vi "GT Pvt Continuous Calculate.vi"(0 "cardNum":i16, 1 "n":i32, 2 "pPos":dbl, 3 "pVel":dbl, 4 "pPercent":dbl, 5 "pVelMax":dbl, 6 "pAcc":dbl, 7 "error in (no error)":errorcluster caption="错误输入（无错误）", 8 "pDec":dbl, 9 "pTime":dbl) -> (18 "pDec out":dbl, 19 "pTime out":dbl, 20 "function return":i16, 22 "pPos out":dbl, 23 "pVel out":dbl, 24 "pPercent out":dbl, 25 "pVelMax out":dbl, 26 "pAcc out":dbl, 27 "error out":errorcluster caption="错误输出")   [LabVIEW 2020, in "gts.lvlib"]
doc: "GT_API GT_PvtContinuousCalculate(short cardNum,long n,double *pPos,double *pVel,double *pPercent,double *pVelMax,double *pAcc,double *pDec,double *pTime);"
uses:
  gts.lvlib
  dll/32bit/multi_card/gts.dll
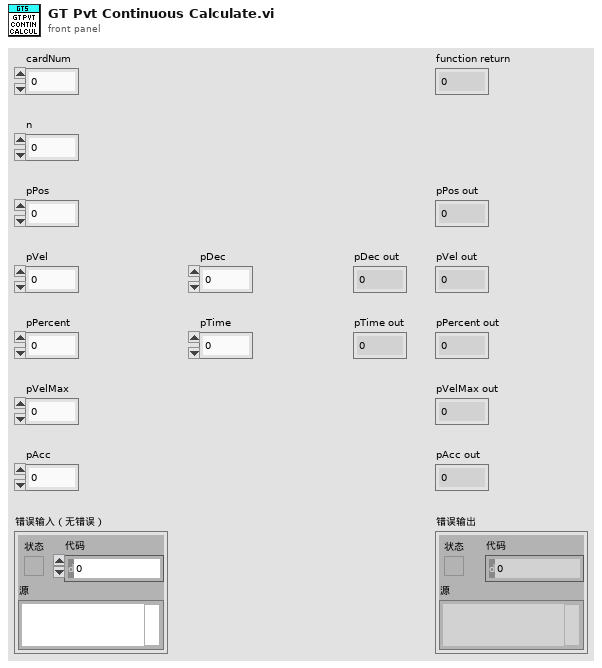
[diagram p1: front panel]
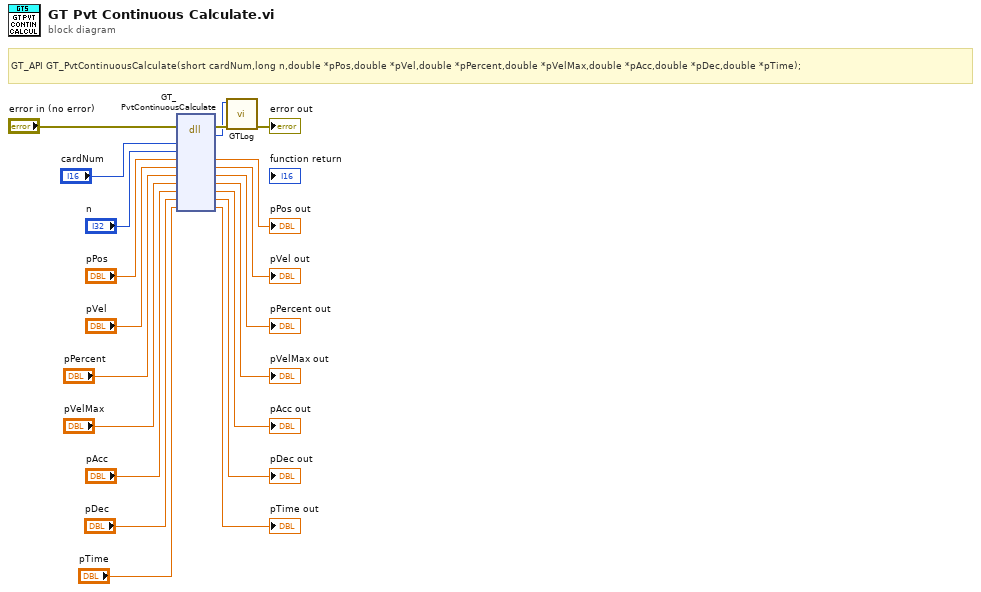
[diagram p0: block diagram]
diagram:
  # "GT_API GT_PvtContinuousCalculate(short cardNum,long n,double *pPos,double *pVel,double *pPercent,double *pVelMax,double *pAcc,double *pDec,double *pTime);"
  n1 = dll-call lib="C:/1228/dll/32bit/multi_card/gts.dll" fn="GT_PvtContinuousCalculate"(error in="error in (no error)", "cardNum"="cardNum", "n"="n", "pPos"="pPos", "pVel"="pVel", "pPercent"="pPercent", "pVelMax"="pVelMax", "pAcc"="pAcc", "pDec"="pDec", "pTime"="pTime") -> (error out=w3:errorcluster, w1:i16, "pPos"=→"pPos out":dbl, "pVel"=→"pVel out":dbl, "pPercent"=→"pPercent out":dbl, "pVelMax"=→"pVelMax out":dbl, "pAcc"=→"pAcc out":dbl, "pDec"=→"pDec out":dbl, "pTime"=→"pTime out":dbl)  [unwired: 4 in, 1 out]
  n2 = call "GTLog.vi"("error in (no error)"=w3, "Numeric"=w1) -> ("error out"=→"error out":errorcluster)  [unwired: 9 in]
